vi "dequeue_state.vi"(7 "stop":bool, 8 "error in (no error)":errorcluster, 11 "queue in":refnum<queue>) -> (0 "error out":errorcluster, 2 "state":T1=enum."(qsm) initialize", 3 "queue out":refnum<queue>)   [LabVIEW 2016]
uses:
  type defs/state.ctl
  type defs/task.ctl
panel:
  # "dequeue_state"
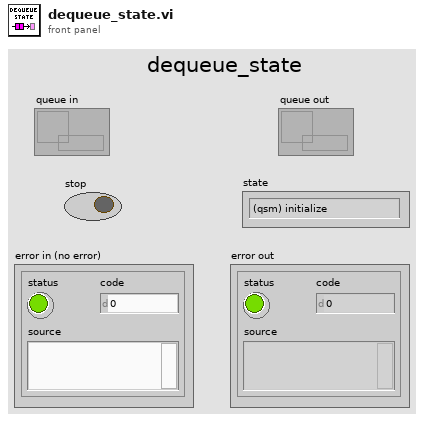
[diagram p1: front panel]
types:
  T1 = typedef "state.ctl" = enum16{"(qsm) schedule", "(qsm) initialize", "(qsm) release", "(qsm) clean up", "(qsm) shutdown", "(myRIO) initialize", "(myRIO) clean up", "(myRIO) update ports", "(image) get", "(image) analyze", "(image) overlay", "(image) show", "save image", "state A", "state B", "state C", "state D", "state E", "state F", "state G", "state H"}
  T2 = typedef "task.ctl" = T1[]
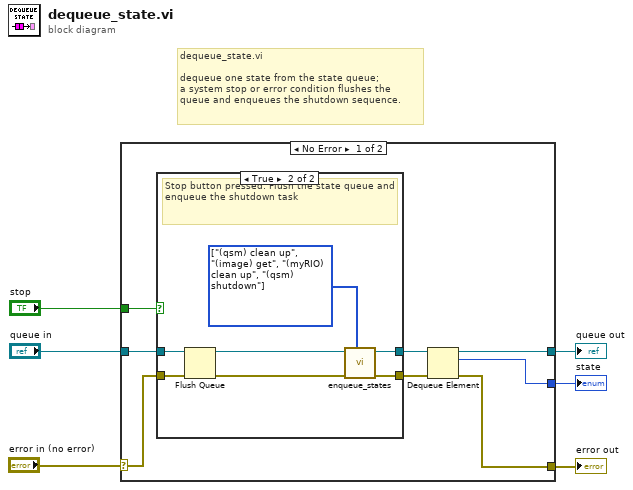
[diagram p0: block diagram]
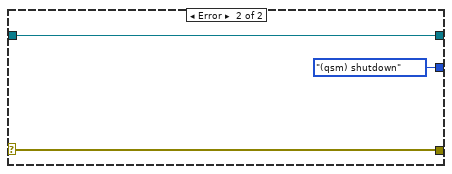
[diagram p3: hidden frame]
diagram:
  # "dequeue_state.vi\n\ndequeue one state from the state queue;\na system stop or error condition flushes the\nqueue and enqueues the shutdown sequence."
  n1 = case shown="No Error" "error in (no error)" {
    selector: "error in (no error)" -> [w7 w24]
    tunnel: "stop" -> [w8 _]
    tunnel: "queue in" -> [w14 w26]
    tunnel: [w11 w24] -> w4
    tunnel: [w10 state."(qsm) shutdown" ("state")] -> w3
    tunnel: [w9 w26] -> w2
    frame No Error {
      n2 = case shown="True" w8 {
        tunnel: w7 -> [w16 w23]
        tunnel: [w16 w20] -> w13
        tunnel: w14 -> [w15 w22]
        tunnel: [w15 w17] -> w12
        frame False {
        }
        frame True {
          w19 = T2 [enum."(qsm) clean up", enum."(image) get", enum."(myRIO) clean up", enum."(qsm) shutdown"] items=["(qsm) schedule", "(qsm) initialize", "(qsm) release", "(qsm) clean up", "(qsm) shutdown", "(myRIO) initialize", "(myRIO) clean up", "(myRIO) update ports", "(image) get", "(image) analyze", "(image) overlay", "(image) show", "save image", "state A", "state B", "state C", "state D", "state E", "state F", "state G", "state H"] ("task")
          # "Stop button pressed: Flush the state queue and enqueue the shutdown task"
          n3 = Flush Queue(queue=w22, error in (no error)=w23) -> (queue out=w18:refnum<queue>, error out=w21:errorcluster)  [unwired: 1 out]
          n4 = call "enqueue_states.vi"("task"=w19, "error in"=w21, "queue in"=w18) -> ("error out"=w20:errorcluster, "queue out"=w17:refnum<queue>)  [unwired: 6 in]
        }
      }
      n5 = Dequeue Element(queue=w12, error in (no error)=w13) -> (queue out=w9:refnum<queue>, element=w10:T1, error out=w11:errorcluster)  [unwired: 1 in, 1 out]
    }
    frame Error {
    }
  }
  "error out" <- w4
  "queue out" <- w2
  "state" <- w3
